vi "VI Tree - error__ogtk.vi"   [LabVIEW 2009]
uses:
  Filter Error Codes (Array)__ogtk.vi
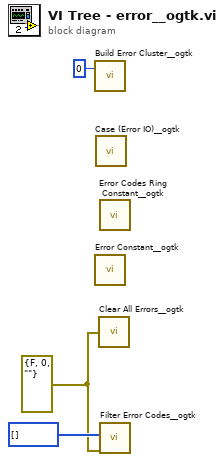
[diagram p0: block diagram]
diagram:
  w1 = errorcluster {"status"=FALSE, "code"=0, "source"=""} ("error in")
  n1 = call "Build Error Cluster__ogtk.vi"("code"=0) -> ()  [unwired: 1 in, 1 out]
  n2 = call "Error Constant__ogtk.vi"() -> ()  [unwired: 1 in]
  n3 = call "Case (Error IO)__ogtk.vi"() -> ()  [unwired: 1 in]
  n4 = call "Clear All Errors__ogtk.vi"("Error In"=w1) -> ()  [unwired: 3 in, 1 out]
  n5 = call "Error Codes Ring Constant__ogtk.vi"() -> ()  [unwired: 1 in]
  n6 = call-poly "Filter Error Codes__ogtk.vi"("Error In"=w1, "Error Codes to Filter"=i32[] [] ("error codes to filter")) -> ()  [unwired: 7 in, 3 out]
